vi "new.vi"() -> ()   [LabVIEW 2020]
panel:
  in  "write buffer":string
  out "read buffer":string
  out "error out":errorcluster
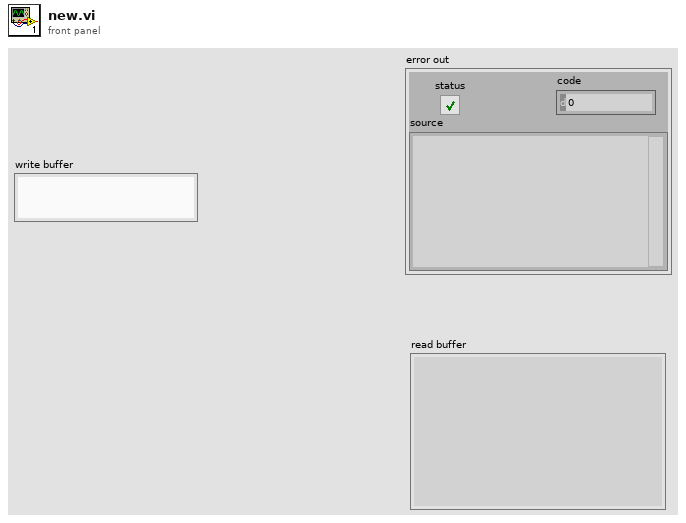
[diagram p1: front panel]
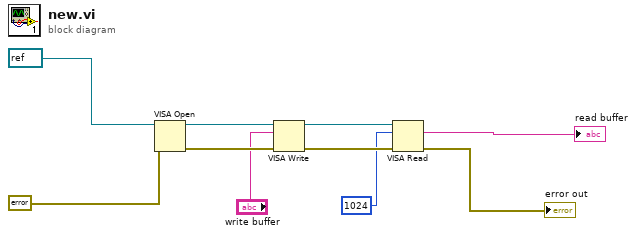
[diagram p0: block diagram]
diagram:
  n1 = VISA Open(error in (no error)=errorcluster {"status"=FALSE, "code"=0, "source"=""}, VISA resource name=refnum<visa-resource-name> refnum) -> (VISA resource name=w8:refnum<visa-resource-name>, error out=w6:errorcluster)  [unwired: 3 in]
  n2 = VISA Write(VISA resource name=w8, write buffer="write buffer", error in (no error)=w6) -> (VISA resource name out=w7:refnum<visa-resource-name>, error out=w5:errorcluster)  [unwired: 1 out]
  n3 = VISA Read(VISA resource name=w7, byte count=u32 1024, error in (no error)=w5) -> (read buffer=→"read buffer":string, error out=→"error out":errorcluster)  [unwired: 2 out]
